vi "Get Byte Order.vi"(11 "Buffer in":refnum<class "Buffer.lvclass">) -> (2 "byte order":T1(ring), 3 "Buffer out":refnum<class "Buffer.lvclass">)   [LabVIEW 2017, in "DSF Core.lvlib" / "Buffer.lvclass"]
uses:
  Buffer.lvclass
  Buffer.lvclass/Buffer.ctl
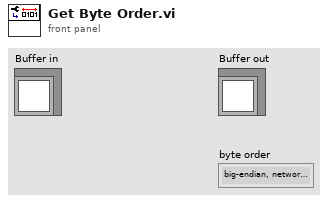
[diagram p1: front panel]
types:
  T1 = enum16{"big-endian, network order", "native, host order", "little-endian"}
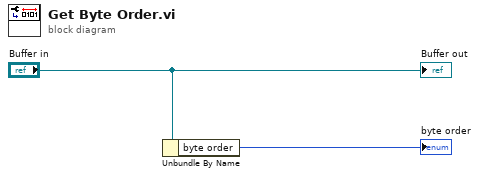
[diagram p0: block diagram]
diagram:
  n1 = Unbundle By Name("Buffer in") -> ("byte order"=→"byte order":T1)
  "Buffer out" <- "Buffer in"
